vi "DetachButton.vi"(4 "pState 2":T1, 5 "Enum":enum16{"Button", "ThumbL", "ThumbR", "Trigger"}(ring)) -> (0 "Trigger":cluster{"Left":bool, "Right":bool}, 1 "Button2":T2, 2 "Thump":T2)   [LabVIEW 2017]
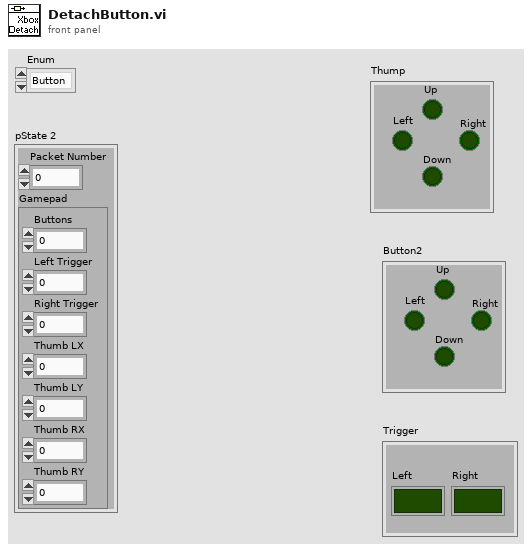
[diagram p1: front panel]
types:
  T1 = cluster{"Packet Number":u32, "Gamepad":cluster{"Buttons":u16, "Left Trigger":u8, "Right Trigger":u8, "Thumb LX":i16, "Thumb LY":i16, "Thumb RX":i16, "Thumb RY":i16}}
  T2 = cluster{"Down":bool, "Up":bool, "Right":bool, "Left":bool}
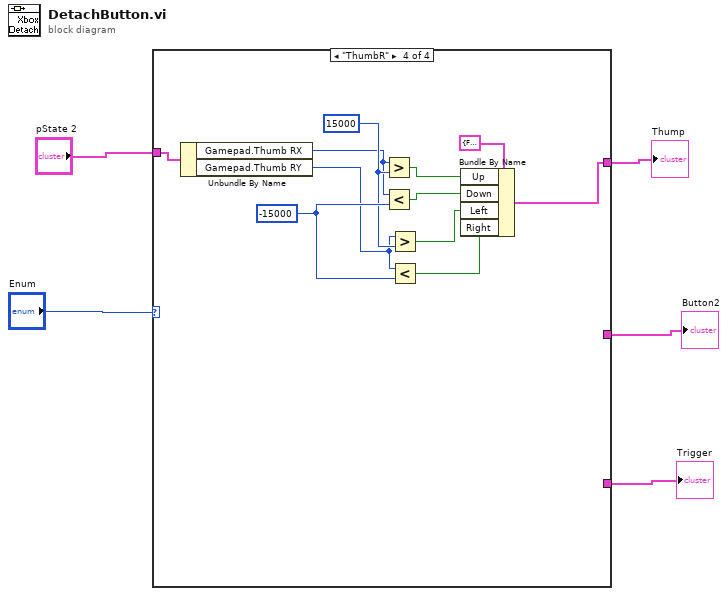
[diagram p0: block diagram]
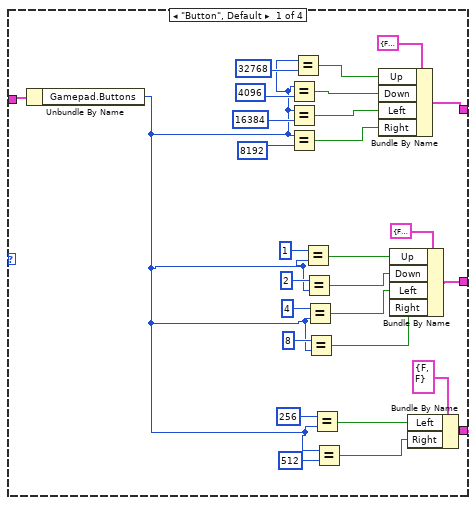
[diagram p2: hidden frame]
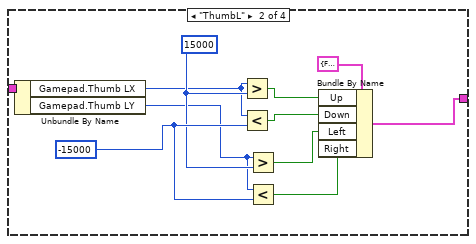
[diagram p3: hidden frame]
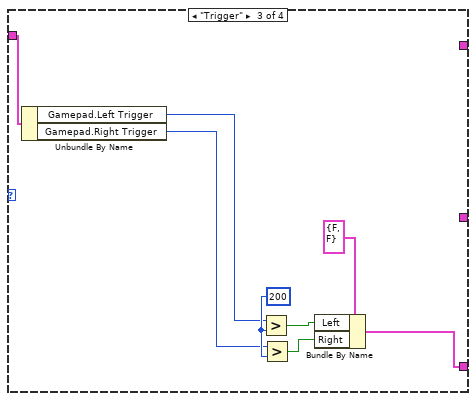
[diagram p4: hidden frame]
diagram:
  n1 = case shown="\"ThumbR\"" "Enum" {
    tunnel: [w29 w43 _ w56] -> w5
    tunnel: [w22 _ _ _] -> w4
    tunnel: [w12 _ w48 _] -> w3
    tunnel: "pState 2" -> [w7 w36 w47 w53]
    frame "Button", Default {
      n2 = Unbundle By Name(w7) -> ("Gamepad.Buttons"=w6:u16)
      n3 = Equal?(x=w6, y=u16 4096) -> (x = y?=w27:bool)
      n4 = Equal?(x=w6, y=u16 16384) -> (x = y?=w26:bool)
      n5 = Equal?(x=w6, y=u16 8192) -> (x = y?=w25:bool)
      n6 = Equal?(x=w6, y=u16 32768) -> (x = y?=w28:bool)
      n7 = Equal?(x=u16 1, y=w6) -> (x = y?=w21:bool)
      n8 = Equal?(x=u16 2, y=w6) -> (x = y?=w20:bool)
      n9 = Equal?(x=u16 4, y=w6) -> (x = y?=w19:bool)
      n10 = Equal?(x=u16 8, y=w6) -> (x = y?=w18:bool)
      n11 = Equal?(x=u16 256, y=w6) -> (x = y?=w11:bool)
      n12 = Equal?(x=w6, y=u16 512) -> (x = y?=w10:bool)
      n13 = Bundle By Name(cluster=T2 {"Down"=FALSE, "Up"=FALSE, "Right"=FALSE, "Left"=FALSE} ("Button2"), "Up"=w28, "Down"=w27, "Left"=w26, "Right"=w25) -> (w29:T2)
      n14 = Bundle By Name(cluster=T2 {"Down"=FALSE, "Up"=FALSE, "Right"=FALSE, "Left"=FALSE} ("Button2"), "Up"=w21, "Down"=w20, "Left"=w19, "Right"=w18) -> (w22:T2)
      n15 = Bundle By Name(cluster=cluster{"Left":bool, "Right":bool} {"Left"=FALSE, "Right"=FALSE} ("Button3"), "Left"=w11, "Right"=w10) -> (w12:cluster{"Left":bool, "Right":bool})
    }
    frame "ThumbL" {
      w37 = 15000
      w40 = -15000
      n16 = Unbundle By Name(w36) -> ("Gamepad.Thumb LX"=w35:i16, "Gamepad.Thumb LY"=w34:i16)
      n17 = Greater?(x=w35, y=w37) -> (0:w42:bool)
      n18 = Less?(x=w35, y=w40) -> (x < y?=w41:bool)
      n19 = Greater?(x=w34, y=w37) -> (0:w39:bool)
      n20 = Less?(x=w34, y=w40) -> (x < y?=w38:bool)
      n21 = Bundle By Name(cluster=T2 {"Down"=FALSE, "Up"=FALSE, "Right"=FALSE, "Left"=FALSE} ("Button2"), "Up"=w42, "Down"=w41, "Left"=w39, "Right"=w38) -> (w43:T2)
    }
    frame "Trigger" {
      w50 = i16 200 ("y")
      n22 = Unbundle By Name(w47) -> ("Gamepad.Left Trigger"=w46:u8, "Gamepad.Right Trigger"=w45:u8)
      n23 = Greater?(x=w46, y=w50) -> (0:w52:bool)
      n24 = Greater?(x=w45, y=w50) -> (0:w51:bool)
      n25 = Bundle By Name(cluster=cluster{"Left":bool, "Right":bool} {"Left"=FALSE, "Right"=FALSE} ("Button3"), "Left"=w52, "Right"=w51) -> (w48:cluster{"Left":bool, "Right":bool})
    }
    frame "ThumbR" {
      w58 = 15000
      w59 = -15000
      n26 = Unbundle By Name(w53) -> ("Gamepad.Thumb RX"=w55:i16, "Gamepad.Thumb RY"=w54:i16)
      n27 = Greater?(x=w55, y=w58) -> (0:w63:bool)
      n28 = Less?(x=w55, y=w59) -> (x < y?=w62:bool)
      n29 = Greater?(x=w54, y=w58) -> (0:w61:bool)
      n30 = Less?(x=w54, y=w59) -> (x < y?=w60:bool)
      n31 = Bundle By Name(cluster=T2 {"Down"=FALSE, "Up"=FALSE, "Right"=FALSE, "Left"=FALSE} ("Button2"), "Up"=w63, "Down"=w62, "Left"=w61, "Right"=w60) -> (w56:T2)
    }
  }
  "Thump" <- w5
  "Button2" <- w4
  "Trigger" <- w3
